vi "Get_Data_With_Condition.vi"(8 "error in (no error)":errorcluster caption="entrée d'erreur (pas d'erreur)", 11 "Firebase Benches en entrée":refnum<class "Firebase Packaging.lvclass">) -> (0 "error out":errorcluster caption="sortie d'erreur", 3 "Firebase Benches en sortie":refnum<class "Firebase Packaging.lvclass">)   [LabVIEW 2020, in "Library Instrument & Equipement.lvlib" / "Library FireBase.lvlib" / "Firebase Packaging.lvclass"]
doc: "Returns data according to Value_To_Find on Collection_to_find Use Nb_To_Read to determine the number to read\nPlease initialise the following values before use the VI\n - Name BDD\n - Value to find\n - API Key\n - Field Filter\n - Field Order\n - Collection_to_find\n\nIf there is no Field order -> Field Order=Field Filter"
uses:
  Firebase Packaging.lvclass
  C:/Users/ngarcin/OneDrive - Altyor/Standard TB/Class/Firebase/Source/Firebase Driver/Firebase Driver.lvclass
  Firebase Packaging.lvclass/Firebase Packaging.ctl
  JSON API/JSON Value/Set from JSON string.vi
  JSON API/JSON Value/JSON Value.lvclass
  Firebase Altyor/Firebase Altyor.lvclass
  JSON API/Variant JSON/Variant JSON.lvlib
  JSON API/Get Polymorphic/JSON GetSet.lvlib
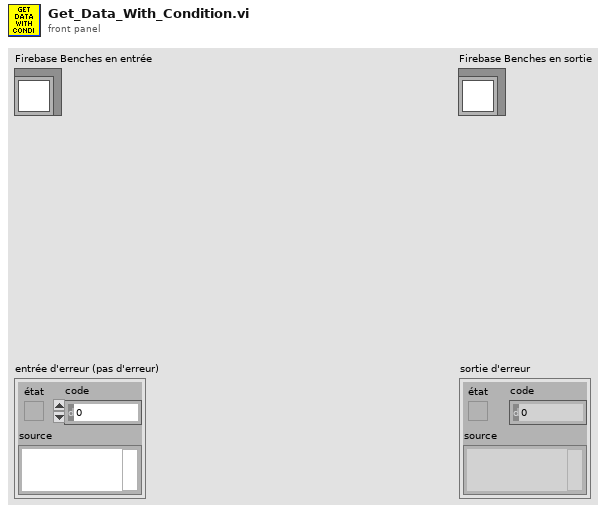
[diagram p1: front panel]
types:
  T1 = cluster{"name":string, "fields":cluster{"Result":cluster{"booleanValue":bool}, "CreationDate":cluster{"timestampValue":string}, "Batch":cluster{"stringValue":string}, "SerialNumber":cluster{"stringValue":string}, "EndOfProduction":cluster{"timestampValue":string}, "PartNumber":cluster{"stringValue":string}, "OrderNumber":cluster{"stringValue":string}, "Operator":cluster{"stringValue":string}}}[]
  T2 = cluster{"name":string, "fields":cluster{"Result":cluster{"booleanValue":bool}, "CreationDate":cluster{"timestampValue":string}, "Batch":cluster{"stringValue":string}, "SerialNumber":cluster{"stringValue":string}, "EndOfProduction":cluster{"timestampValue":string}, "PartNumber":cluster{"stringValue":string}, "OrderNumber":cluster{"stringValue":string}, "Operator":cluster{"stringValue":string}}}
  T3 = cluster{"document":cluster{"name":string, "fields":cluster{"Result":cluster{"booleanValue":bool}, "CreationDate":cluster{"timestampValue":string}, "Batch":cluster{"stringValue":string}, "SerialNumber":cluster{"stringValue":string}, "EndOfProduction":cluster{"timestampValue":string}, "PartNumber":cluster{"stringValue":string}, "OrderNumber":cluster{"stringValue":string}, "Operator":cluster{"stringValue":string}}}}
  T4 = cluster{"document":cluster{"name":string, "fields":cluster{"Result":cluster{"booleanValue":bool}, "CreationDate":cluster{"timestampValue":string}, "Batch":cluster{"stringValue":string}, "SerialNumber":cluster{"stringValue":string}, "EndOfProduction":cluster{"timestampValue":string}, "PartNumber":cluster{"stringValue":string}, "OrderNumber":cluster{"stringValue":string}, "Operator":cluster{"stringValue":string}}}}[]
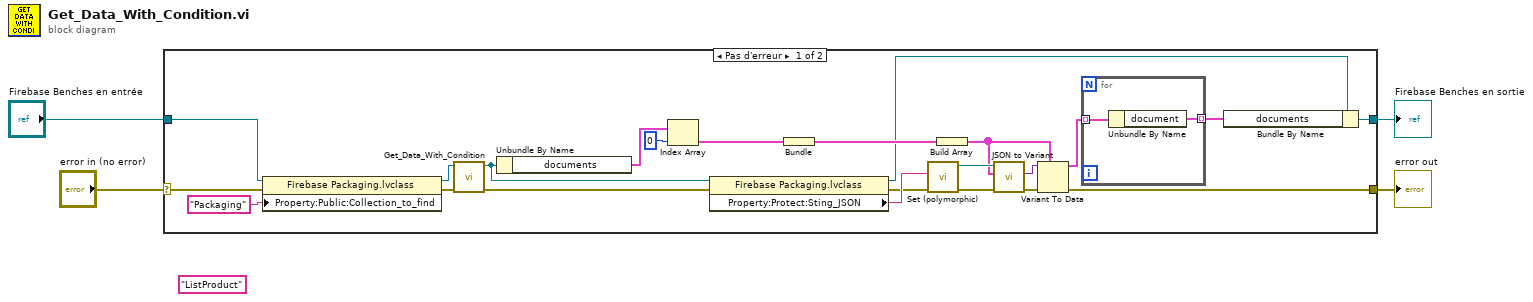
[diagram p0: block diagram]
diagram:
  (unwired) "ListProduct" ("Collection_to_find")
  n1 = case shown="Pas d'erreur" "error in (no error)" {
    selector: "error in (no error)" -> [w6 w31]
    tunnel: "Firebase Benches en entrée" -> [w9 w30]
    tunnel: [w10 w31] -> w3
    tunnel: [w13 w30] -> w2
    frame No Error {
      n2 = property class="Firebase Packaging.lvclass"(reference=w9, error in=w6, "Property:Public:Collection_to_find"="Packaging" ("Collection_to_find")) -> (reference out=w8:refnum<class "Firebase Packaging.lvclass">, error out=w5:errorcluster)
      n3 = call-parent "Get_Data_With_Condition.vi"("error in (no error)"=w5, "Firebase Benches en entrée"=w8) -> ("error out"=w16:errorcluster, "Firebase Benches en sortie"=w15:refnum<class "Firebase Packaging.lvclass">)  [unwired: 8 in]
      n4 = Unbundle By Name(w15) -> ("documents"=w22:T1)
      n5 = Index Array(array=w22, index=0 ("indice")) -> (element=w20:T2)
      n6 = property class="Firebase Packaging.lvclass"(reference=w15, error in=w16) -> (reference out=w12:refnum<class "Firebase Packaging.lvclass">, error out=w14:errorcluster, "Property:Protect:Sting_JSON"=w23:string)
      n7 = Bundle("document"=w20) -> (w19:T3)  [unwired: 1 in]
      n8 = call-poly "Set (polymorphic).vi"("error in (no error)"=w14, "JSON stream"=w23) -> ("error out"=w24:errorcluster, "JSON Value out"=w26:refnum<class "JSON Value.lvclass">)  [unwired: 7 in, 1 out]
      n9 = Build Array(w19) -> (w18:T4)
      n10 = call "JSON to Variant.vi"("error in (no error)"=w24, "Variant (Data Type)"=w18, "JSON Value"=w26) -> ("error out"=w25:errorcluster, "Variant out"=w11:variant)  [unwired: 7 in]
      n11 = Variant To Data(error in=w25, type=w18, Variant=w11) -> (data=w17:T4, error out=w10:errorcluster)
      n12 = for {
        tunnel: w17 -> [w29] mode=indexing
        tunnel: [w28] -> w27 mode=indexing
        n13 = Unbundle By Name(w29) -> ("document"=w28:T2)
      }
      n14 = Bundle By Name(cluster=w12, "documents"=w27) -> (w13:refnum<class "Firebase Packaging.lvclass">)
    }
    frame Error {
    }
  }
  "error out" <- w3
  "Firebase Benches en sortie" <- w2
